vi "Default Supported FileType.vi"() -> (3 "Array":string[](array[string]))   [LabVIEW 2014]
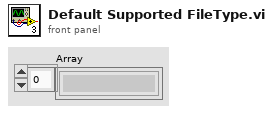
[diagram p1: front panel]
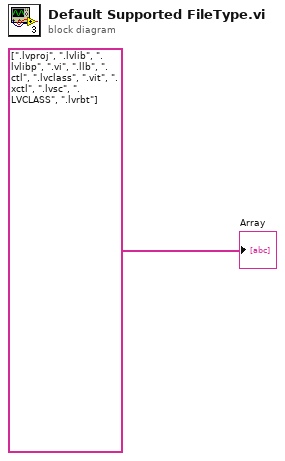
[diagram p0: block diagram]
diagram:
  "Array" <- string[] [".lvproj", ".lvlib", ".lvlibp", ".vi", ".llb", ".ctl", ".lvclass", ".vit", ".xctl", ".lvsc", ".LVCLASS", ".lvrbt"] ("Array")
